vi "Generate CSV Report.vi"(0 "Report Variables":T1, 4 "Lower Limits":dbl[](array[numeric]), 5 "Measurment values":dbl[](array[numeric]), 7 "Upper Limits":dbl[](array[numeric]), 9 "Status":string[](array[string]), 11 "Overall status":string, 13 "Test Names":string[](array[string])) -> (19 "error out":errorcluster)   [LabVIEW 2025]
uses:
  Station/Controls/Report Variables.ctl
  <vilib>/Utility/file.llb/Write Delimited Spreadsheet (string).vi
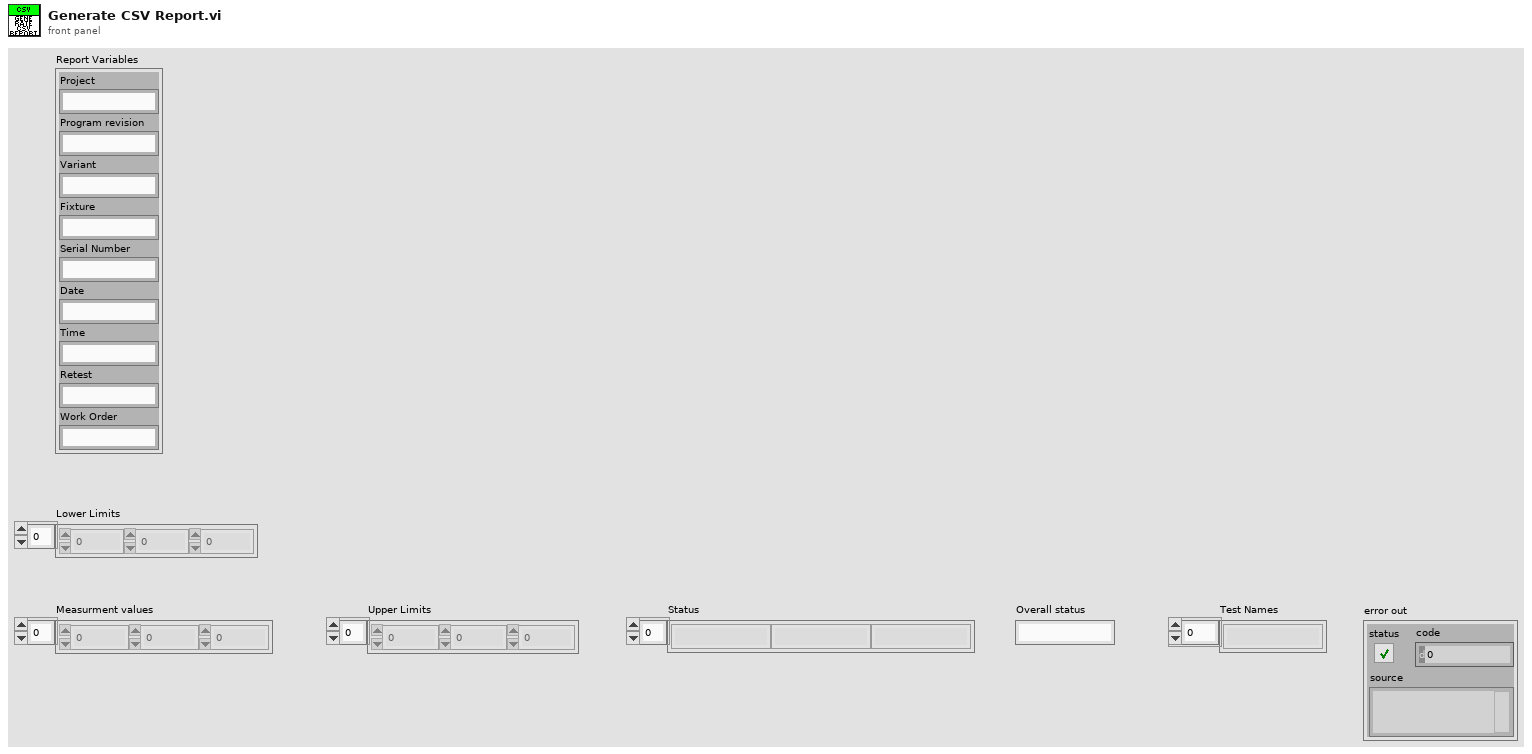
[diagram p1: front panel]
types:
  T1 = typedef "Report Variables.ctl" = cluster{"Project ":string, "Program revision":string, "Variant":string, "Fixture":string, "Serial Number":string, "Date":string, "Time":string, "Retest":string, "Work Order":string}
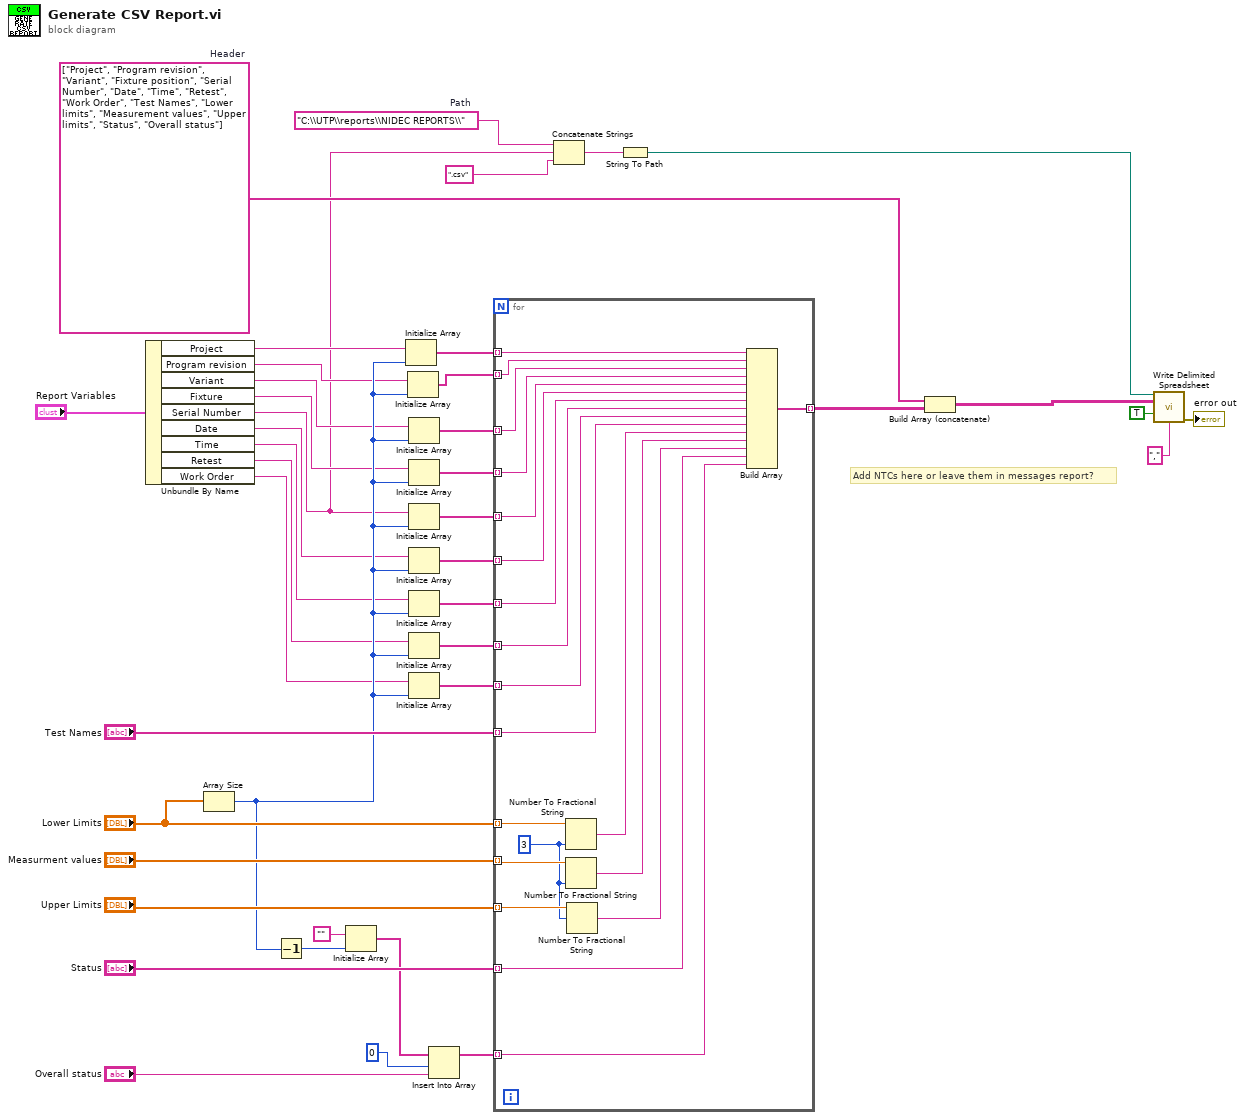
[diagram p0: block diagram]
diagram:
  w25 = "C:\\UTP\\reports\\NIDEC REPORTS\\"  # Path
  w29 = string[] ["Project", "Program revision", "Variant", "Fixture position", "Serial Number", "Date", "Time", "Retest", "Work Order", "Test Names", "Lower limits", "Measurement values", "Upper limits", "Status", "Overall status"]  # Header
  # "Add NTCs here or leave them in messages report?"
  n1 = Unbundle By Name("Report Variables") -> ("Project"=w9:string, "Program revision"=w8:string, "Variant"=w7:string, "Fixture"=w6:string, "Serial Number"=w5:string, "Date"=w4:string, "Time"=w3:string, "Retest"=w2:string, "Work Order"=w1:string)
  n2 = Array Size(array="Lower Limits") -> (size(s)=w11:i32)
  n3 = Decrement(x=w11) -> (x-1=w20:i32)
  n4 = Initialize Array("", w20) -> (w14:string[])
  n5 = Initialize Array(w9, w11) -> (w41:string[])
  n6 = Initialize Array(w8, w11) -> (w12:string[])
  n7 = Initialize Array(w7, w11) -> (w40:string[])
  n8 = Initialize Array(w6, w11) -> (w39:string[])
  n9 = Initialize Array(w5, w11) -> (w30:string[])
  n10 = Initialize Array(w4, w11) -> (w38:string[])
  n11 = Initialize Array(w3, w11) -> (w37:string[])
  n12 = Initialize Array(w2, w11) -> (w26:string[])
  n13 = Initialize Array(w1, w11) -> (w18:string[])
  n14 = Insert Into Array(array=w14, index=0, new element="Overall status") -> (w32:string[])
  n15 = for {
    tunnel: w41 -> [w43] mode=indexing
    tunnel: w40 -> [w56] mode=indexing
    tunnel: w39 -> [w55] mode=indexing
    tunnel: w30 -> [w54] mode=indexing
    tunnel: w38 -> [w53] mode=indexing
    tunnel: w37 -> [w52] mode=indexing
    tunnel: "Lower Limits" -> [w61] mode=indexing
    tunnel: "Measurment values" -> [w60] mode=indexing
    tunnel: "Upper Limits" -> [w59] mode=indexing
    tunnel: "Status" -> [w46] mode=indexing
    tunnel: w32 -> [w44] mode=indexing
    tunnel: [w57] -> w28 mode=indexing
    tunnel: w26 -> [w51] mode=indexing
    tunnel: w18 -> [w50] mode=indexing
    tunnel: "Test Names" -> [w45] mode=indexing
    tunnel: w12 -> [w42] mode=indexing
    w58 = i16 3 ("precision (6)")
    n16 = Number To Fractional String(number=w61, precision (6)=w58) -> (F-format string=w49:string)  [unwired: 2 in]
    n17 = Number To Fractional String(number=w60, precision (6)=w58) -> (F-format string=w48:string)  [unwired: 2 in]
    n18 = Number To Fractional String(number=w59, width (-)=w58) -> (F-format string=w47:string)  [unwired: 2 in]
    n19 = Build Array(w43, w42, w56, w55, w54, w53, w52, w51, w50, w45, w49, w48, w47, w46, w44) -> (w57:string[])
  }
  n20 = Concatenate Strings(w25, w5, ".csv" ("string")) -> (w24:string)
  n21 = String To Path(string=w24) -> (path=w23:path)
  n22 = Build Array (concatenate)(w29, w28) -> (w27:string[][])
  n23 = call-poly <vilib>:"Write Delimited Spreadsheet.vi"("file path (dialog if empty)"=w23, "2D data"=w27, "append to file? (new file:F)"=TRUE, "delimiter (\\t)"="," ("delimiter (\\t)")) -> ("error out"=→"error out":errorcluster)  [unwired: 10 in, 1 out]
